vi "Find camera co-ordinate.vi"(10 "Read cam":string="1,3.644,3.358,7.44,7.546") -> (1 "RSTC":string, 2 "length":i32, 3 "RSBC":string, 4 "RBT":string, 5 "ok/ng":string, 6 "LBT":string)   [LabVIEW 2020]
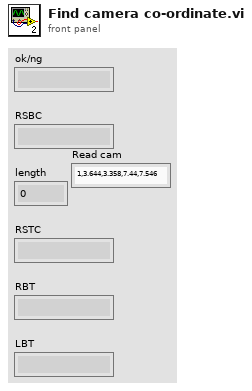
[diagram p1: front panel]
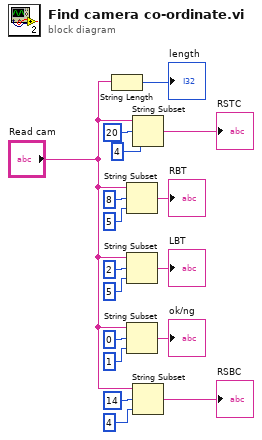
[diagram p0: block diagram]
diagram:
  n1 = String Length(string="Read cam") -> (length=→"length":i32)
  n2 = String Subset(string="Read cam", offset (0)=8, length (rest)=5 ("length (rest)")) -> (substring=→"RBT":string)
  n3 = String Subset(string="Read cam", offset (0)=2, length (rest)=5 ("length (rest)")) -> (substring=→"LBT":string)
  n4 = String Subset(string="Read cam", offset (0)=0, length (rest)=1 ("length (rest)")) -> (substring=→"ok/ng":string)
  n5 = String Subset(string="Read cam", offset (0)=20, length (rest)=4 ("length (rest)")) -> (substring=→"RSTC":string)
  n6 = String Subset(string="Read cam", offset (0)=14, length (rest)=4 ("length (rest)")) -> (substring=→"RSBC":string)
